vi "EvaluateTriggerConditions.vi"(8 "error in (no error)":errorcluster, 9 "data":T1, 10 "config in":T5, 11 "Qbus in":refnum<class "Qbus.lvclass">) -> (0 "error out":errorcluster, 2 "config out":T5, 3 "Qbus out":refnum<class "Qbus.lvclass">)   [LabVIEW 2017, in "Trigger.lvlib"]
uses:
  <vilib>/addons/InsightCM/Devices/Shared/Common/Trigger/Trigger.lvlib
  <vilib>/addons/InsightCM/Devices/Shared/Common/Trigger/controls/config.ctl
  <vilib>/addons/Qbus/Qbus.lvclass
  <vilib>/addons/InsightCM/Devices/Shared/Common/DataFlow/controls/Data.ctl
  <vilib>/addons/InsightCM/Utilities/DataAccessors/controls/wfmSGL_DVR.ctl
  <vilib>/addons/PointValueMap/controls/PointMap.ctl
  <vilib>/addons/InsightCM/Devices/Shared/Common/DataFlow/controls/Type.ctl
  <vilib>/addons/InsightCM/Devices/Shared/Common/Trigger/controls/ConditionType.ctl
  <vilib>/addons/PointValueMap/subVIs/Point_Read_string.vi
  <vilib>/addons/PointValueMap/subVIs/Point_Write_string.vi
  <vilib>/addons/PointValueMap/PointValueMap.lvlib
  <vilib>/addons/InsightCM/Devices/Shared/Common/DataFlow/DataFlow.lvlib
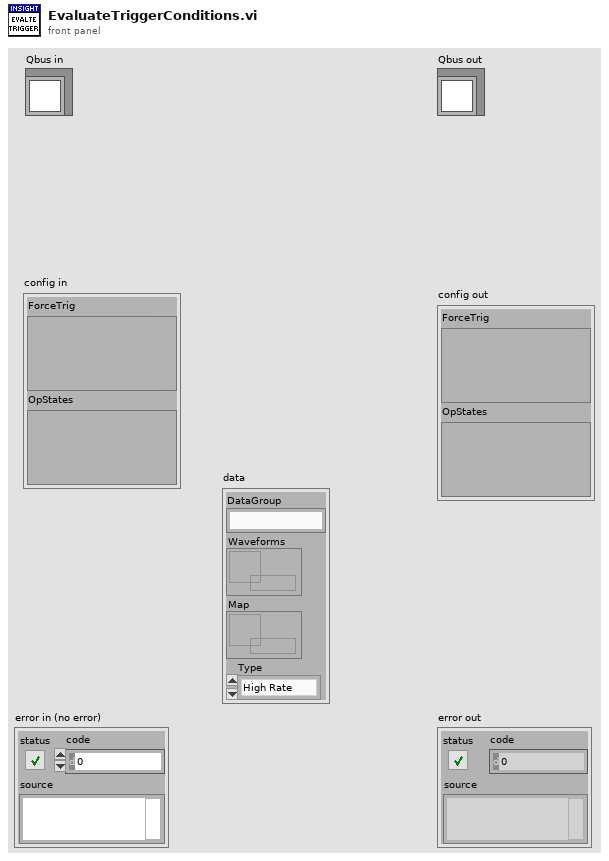
[diagram p1: front panel]
types:
  T1 = typedef "DataFlow.lvlib/Data.ctl" = cluster{"DataGroup":string, "Waveforms":T2, "Map":T3, "Type":T4}
  T2 = typedef "wfmSGL_DVR.ctl" = refnum<data-value>
  T3 = typedef "PointValueMap.lvlib/PointMap.ctl" = refnum<data-value>
  T4 = typedef "DataFlow.lvlib/Type.ctl" = enum16{"High Rate", "Low Rate", "Burst Mode"}
  T5 = typedef "Trigger.lvlib/config.ctl" = cluster{"ForceTrig":variant, "OpStates":variant}
  T6 = typedef "Trigger.lvlib/ConditionType.ctl" = enum16{"FileCollection", "TrendCollection"}
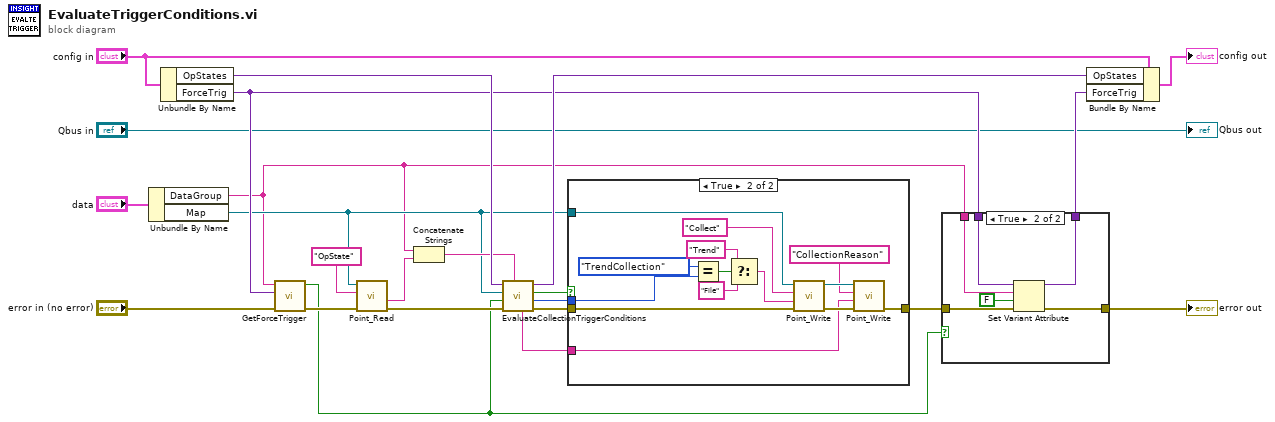
[diagram p0: block diagram]
diagram:
  n1 = Unbundle By Name("data") -> ("DataGroup"=w4:string, "Map"=w5:T3)
  n2 = Unbundle By Name("config in") -> ("OpStates"=w21:variant, "ForceTrig"=w17:variant)
  n3 = call <vilib>:"GetForceTrigger.vi"("error in"="error in (no error)", "status"=w17, "data group"=w4) -> ("error out"=w11:errorcluster, "force trigger"=w1:bool)  [unwired: 7 in]
  n4 = call-poly <vilib>:"Point_Read.vi"("Error In"=w11, "Tag"="OpState", "Map"=w5) -> ("Error Out"=w10:errorcluster, "Value"=w9:string)  [unwired: 3 in, 4 out]
  n5 = Concatenate Strings(w4, w9) -> (w8:string)
  n6 = call <vilib>:"EvaluateCollectionTriggerConditions.vi"("dg_opState"=w8, "error in"=w10, "force trigger"=w1, "map"=w5, "OpStates in"=w21) -> ("error out"=w7:errorcluster, "collection type"=w2:T6, "collect"=w3:bool, "OpStates out"=w18:variant, "reason"=w16:string)  [unwired: 2 in]
  n7 = case shown="True" w3 {
    tunnel: w7 -> [w24 w38]
    tunnel: w16 -> [_ w32]
    tunnel: [w24 w35] -> w14
    tunnel: w5 -> [_ w34]
    tunnel: w2 -> [_ w29]
    frame False {
    }
    frame True {
      n8 = Equal?(x=ConditionType."TrendCollection", y=w29) -> (x = y?=w28:bool)
      n9 = Select(t="Trend" ("Tag"), s=w28, f="File" ("Tag")) -> (s? t:f=w26:string)
      n10 = call-poly <vilib>:"Point_Write.vi"("Error In"=w38, "Value"=w26, "Tag"="Collect", "Map"=w34) -> ("Error Out"=w37:errorcluster, "Map Out"=w36:T3)  [unwired: 6 in]
      n11 = call-poly <vilib>:"Point_Write.vi"("Error In"=w37, "Value"=w32, "Tag"="CollectionReason", "Map"=w36) -> ("Error Out"=w35:errorcluster)  [unwired: 6 in, 1 out]
    }
  }
  n12 = case shown="True" w1 {
    tunnel: [w39 w46] -> w20
    tunnel: [w40 w45] -> w19
    tunnel: w17 -> [w39 w44]
    tunnel: w14 -> [w40 w43]
    tunnel: w4 -> [_ w42]
    frame False {
    }
    frame True {
      n13 = Set Variant Attribute(Variant=w44, name=w42, value=FALSE, error in=w43) -> (Variant out=w46:variant, error out=w45:errorcluster)  [unwired: 1 out]
    }
  }
  "error out" <- w19
  n14 = Bundle By Name(cluster="config in", "OpStates"=w18, "ForceTrig"=w20) -> (→"config out":T5)
  "Qbus out" <- "Qbus in"
